vi "Test Schnittpunkte_kreis.vi"() -> ()   [LabVIEW 2019]
uses:
  Kreisquadrant/Kreisquadrant.lvclass
  mode_Q.ctl
panel:
  in  "Radius":dbl=10.0
  in  "Sektor":T1(ring)
  out "Sensor auf Linie":bool
  out "Schnittpunkt":dbl[](array[numeric])
  out "XY Graph":cluster{"x":dbl[], "y":dbl[]}[](graph)=[{"x"=[], "y"=[]}, {"x"=[7.0, 14.0], "y"=[0.0, 1.0]}, {"x"=[0.0], "y"=[0.0]}]
  in  "Sensorkoord [P1 P2]":dbl[][](array[numeric])=[[7.0, 14.0], [0.0, 1.0]]
  in  "Zentrum":dbl[](array[numeric])=[10.0, 0.0]
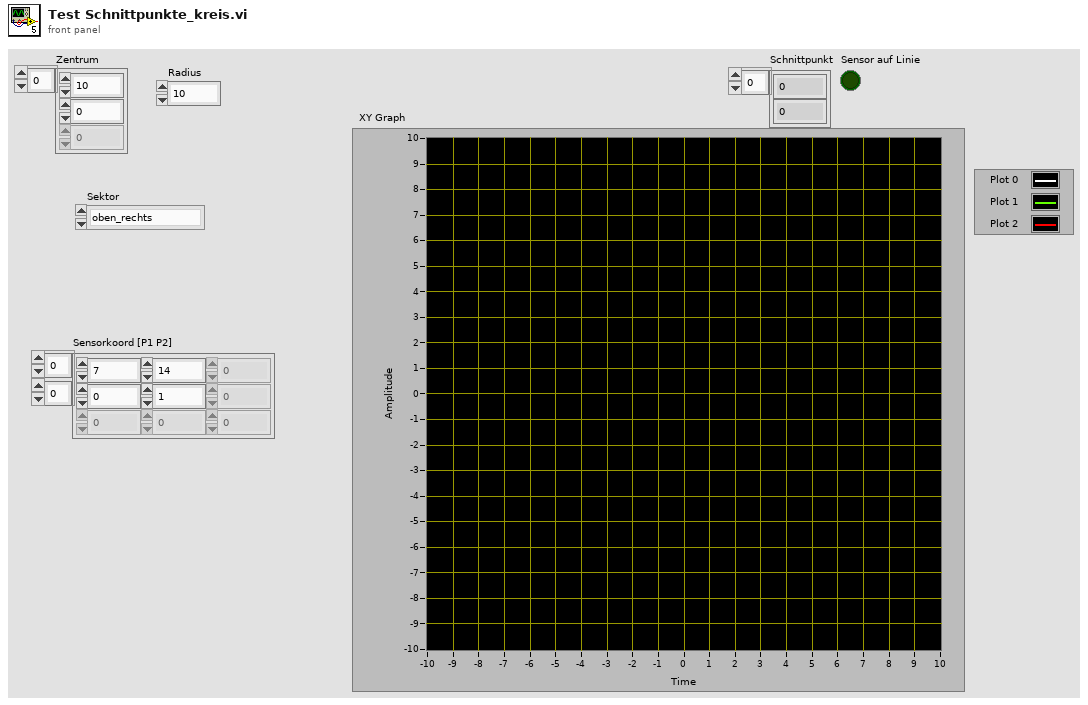
[diagram p1: front panel]
types:
  T1 = enum16{"oben_rechts", "oben_links", "unten_links", "unten_rechts"}
  T2 = typedef "mode_Q.ctl" = enum16{"init", "get"}
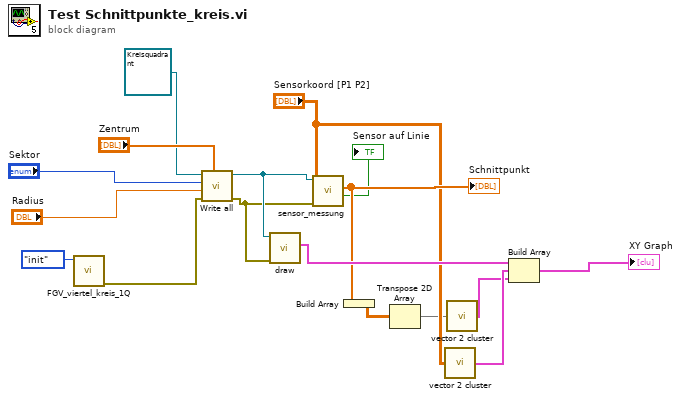
[diagram p0: block diagram]
diagram:
  n1 = call "FGV_viertel_kreis_1Q.vi"("mode"=mode_Q."init") -> ("error out"=w1:errorcluster)  [unwired: 8 in, 2 out]
  n2 = call-dynamic "Write all.vi"("Zentrum"="Zentrum", "error in (no error)"=w1, "Radius"="Radius", "Sektor"="Sektor", "Kreisquadrant in"=refnum<class "Kreisquadrant.lvclass"> refnum) -> ("error out"=w16:errorcluster, "Kreisquadrant out"=w17:refnum<class "Kreisquadrant.lvclass">)  [unwired: 5 in]
  n3 = call-dynamic "draw.vi"("error in (no error)"=w16, "Kreisquadrant in"=w17) -> ("element"=w15:cluster{"x":dbl[], "y":dbl[]})  [unwired: 7 in, 2 out]
  n4 = call-dynamic "sensor_messung.vi"("error in (no error)"=w16, "Sensorkoord [P1 P2]"="Sensorkoord [P1 P2]", "Kreisquadrant in"=w17) -> ("Sensor auf Linie"=→"Sensor auf Linie":bool, "Schnittpunkt"=w13:dbl[])  [unwired: 5 in, 2 out]
  "Schnittpunkt" <- w13
  n5 = Build Array(w13) -> (w12:dbl[][])
  n6 = Transpose 2D Array(2D array=w12) -> (transposed array=w7:dbl[][])
  n7 = call "vector 2 cluster.vi"("coordinates"="Sensorkoord [P1 P2]") -> (0:w9:cluster{"x":dbl[], "y":dbl[]})
  n8 = call "vector 2 cluster.vi"("coordinates"=w7) -> (0:w8:cluster{"x":dbl[], "y":dbl[]})
  n9 = Build Array(w15, w9, w8) -> (→"XY Graph":cluster{"x":dbl[], "y":dbl[]}[])
